vi "New TSD Values.vi"(8 "Error In":errorcluster, 10 "Offset":dbl, 11 "X factor":dbl) -> (0 "Error Out":errorcluster, 2 "Offset out":dbl, 3 "X factor out":dbl)   [LabVIEW 2019, in "GUI.lvlib"]
uses:
  GUI.lvlib
panel:
  out "Current Offset":dbl
  out "Current X factor":dbl
  in  "Cancel Button":bool
  in  "OK Button":bool
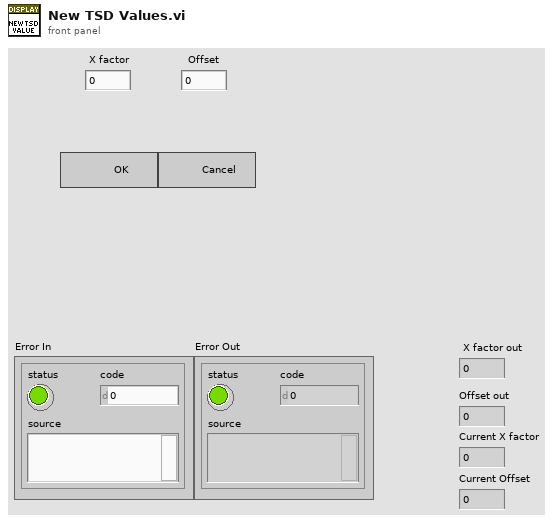
[diagram p1: front panel]
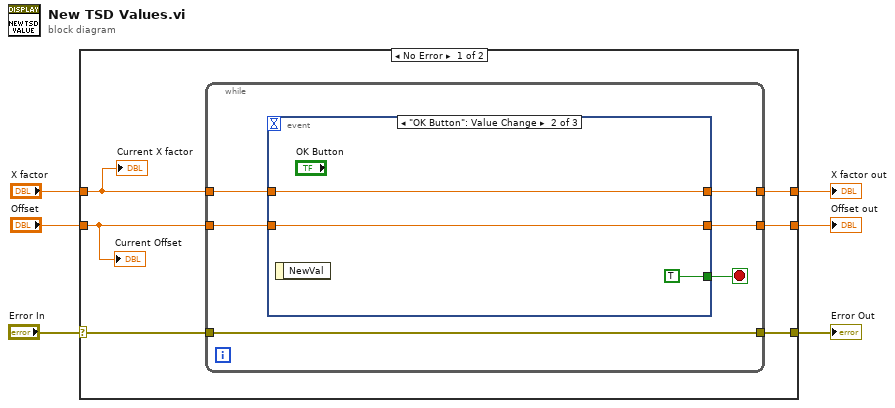
[diagram p0: block diagram]
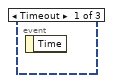
[diagram p2: hidden frame]
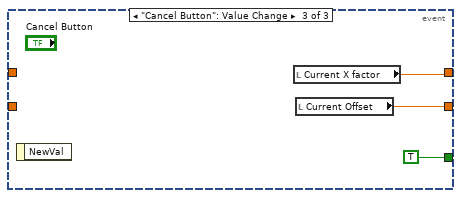
[diagram p3: hidden frame]
diagram:
  n1 = case shown="No Error" "Error In" {
    selector: "Error In" -> [w8 w27]
    tunnel: [w7 w27] -> w5
    tunnel: "X factor" -> [w10 w26]
    tunnel: "Offset" -> [w9 w25]
    tunnel: [w12 w26] -> w2
    tunnel: [w11 w25] -> w1
    frame No Error {
      n2 = while {
        tunnel: w10 -> [w17]
        tunnel: w9 -> [w18]
        tunnel: [w16] -> w12
        tunnel: [w15] -> w11
        tunnel: [w13] -> w7
        tunnel: w8 -> [w13]
        stop <- w14 stop-if-true
        n3 = event shown="[1] \"OK Button\": Value Change" {
          selector: _ -> [_ _ _]
          dyn-events: _ -> [_ _ _]
          timeout: _ -> [_ _ _]
          tunnel: w18 -> [_ w20 _]
          tunnel: w17 -> [_ w21 _]
          tunnel: [_ w21 w24] -> w16
          tunnel: [_ w20 w23] -> w15
          tunnel: [_ TRUE TRUE] -> w14
          event Timeout {
            n4 = event-data() -> ()  [unwired: 1 in, 1 out]
          }
          event "OK Button": Value Change {
            n5 = event-data() -> ()  [unwired: 1 in, 1 out]
          }
          event "Cancel Button": Value Change {
            n6 = event-data() -> ()  [unwired: 1 in, 1 out]
            n7 = local read "Current X factor"() -> (w24:dbl)
            n8 = local read "Current Offset"() -> (w23:dbl)
          }
        }
      }
      "Current X factor" <- w10
      "Current Offset" <- w9
    }
    frame Error {
    }
  }
  "Error Out" <- w5
  "X factor out" <- w2
  "Offset out" <- w1
